vi "Temp_read.vi"() -> ()   [LabVIEW 2020]
panel:
  in  "group name in":string="Data"
  in  "channel name(s) in":string[](array[string])
  out "data":waveform(dbl)[](array[waveform])
  in  "base path":path
  in  "name or relative path":path
  in  "file format version (2.0)":enum16{"1.0", "2.0"}(ring)
  in  "operation (0:open)":T1(ring)=enum."open or create"
  out "error out":errorcluster
  in  "stop":bool
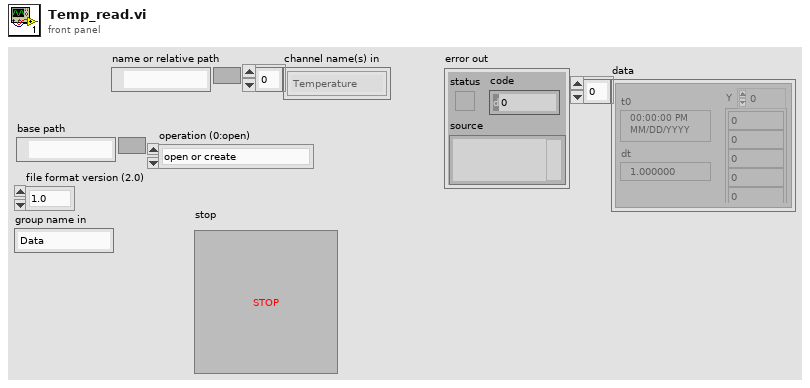
[diagram p1: front panel]
types:
  T1 = enum16{"open", "open or create", "create or replace", "create", "open (read-only)"}
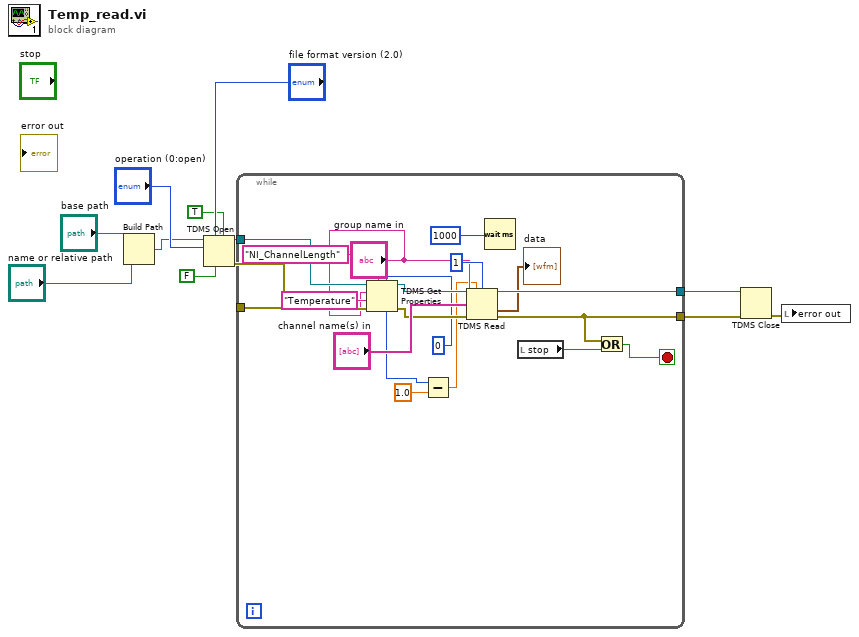
[diagram p0: block diagram]
diagram:
  n1 = Build Path(base path="base path", name or relative path="name or relative path") -> (appended path=w3:path)
  n2 = TDMS Open(5:TRUE ("create index file? (T)"), 6:FALSE ("disable buffering? (T)"), 7:"file format version (2.0)", 10:"operation (0:open)", 11:w3) -> (0:w7:errorcluster, 3:w10:refnum<k34>)  [unwired: 2 in]
  n3 = while {
    tunnel: w10 -> [w23]
    tunnel: [w30] -> w9
    tunnel: [w28] -> w8
    tunnel: w7 -> [w20]
    stop <- w27 stop-if-true
    n4 = TDMS Get Properties(5:0, 7:"NI_ChannelLength" ("property name"), 8:w20, 9:"Temperature" ("channel name"), 10:"group name in", 11:w23) -> (0:w21:errorcluster, 3:w22:refnum<k34>, 4:w14:i32)  [unwired: 3 out]
    n5 = Subtract(x=w14, y=1.0) -> (x-y=w13:dbl)
    n6 = TDMS Read(0:w22, 1:w13, 2:i64 1 ("count (-1: all)"), 5:"group name in", 7:"channel name(s) in", 11:w21) -> (4:w30:refnum<k34>, 10:→"data":waveform(dbl)[], 15:w28:errorcluster)  [unwired: 2 in, 3 out]
    n7 = Wait (ms)(milliseconds to wait=u32 1000) -> ()  [unwired: 1 out]
    n8 = local read "stop"() -> (w29:bool)
    n9 = Or(x=w28, y=w29) -> (x .or. y?=w27:bool)
  }
  n10 = TDMS Close(8:w8, 11:w9) -> (0:w6:errorcluster)  [unwired: 1 out]
  n11 = local write "error out"(w6) -> ()
